vi "XIPIN_3GPP_RACH_Preamble_Detector_1_0.vi"   [LabVIEW 2017]
doc: "The 3GPP RACH Preamble Detector core provides an optimal solution for implementing RACH detection in a 3GPP uplink. The core includes all of the logic required for scramble-code generation, correlation and preamble detection. The RACH Preamble Detector combines an optimal core and a flexible wrapper design.\n------------------------------------\n<b>Need License</b> : Yes"
uses:
  <vilib>/rvi/XilinxIP/XIPIN_XNode/niFpgaXIPIN.xnode
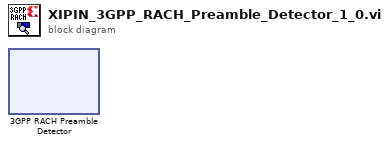
[diagram p0: block diagram]
diagram:
  n1 = xnode ("3GPP RACH Preamble Detector")() -> ()
